vi "movimento.vi"(9 "Condição de parada":bool=TRUE, 10 "Motor speed":i32=60, 11 "Direção":T1(ring)) -> ()   [LabVIEW 2016]
uses:
  <vilib>/NXT/Block Support/NXT_InputPort.ctl
  <vilib>/NXT/Block Support/NXT_OutputPort.ctl
  <vilib>/NXT/Dual Mode Library/Sensors/EV3_Gyro_Reset.vi
  <vilib>/NXT/Dual Mode Library/Sensors/EV3_Gyro_Angle.vi
  <vilib>/NXT/NXTIO Xnodes/NXTIONodeSubVIs/NXTMoveMotors.vi
  <vilib>/NXT/NXTIO Xnodes/NXTIONodeSubVIs/NXTStopMotors.vi
  <vilib>/NXT/Subs/LVHSConnector.ctl
  <vilib>/NXT/NXTIO Xnodes/AddressXNode/NXTIOAddress.xnode
  <vilib>/NXT/NXTIO Xnodes/NXTIOXNode/NXTIO.xnode
  <vilib>/NXT/LegoClasses/BrickReference/BrickReference.lvclass
panel:
  out "Degrees":sgl
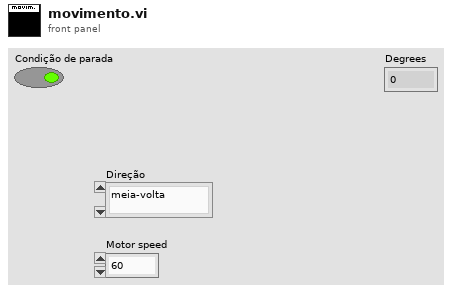
[diagram p1: front panel]
types:
  T1 = enum16{"meia-volta", "esquerda", "direita", "frente"}
  T2 = typedef "NXT_InputPort.ctl" = u32
  T3 = typedef "LVHSConnector.ctl" = refnum<class "BrickReference.lvclass">
  T4 = typedef "NXT_OutputPort.ctl" = u8
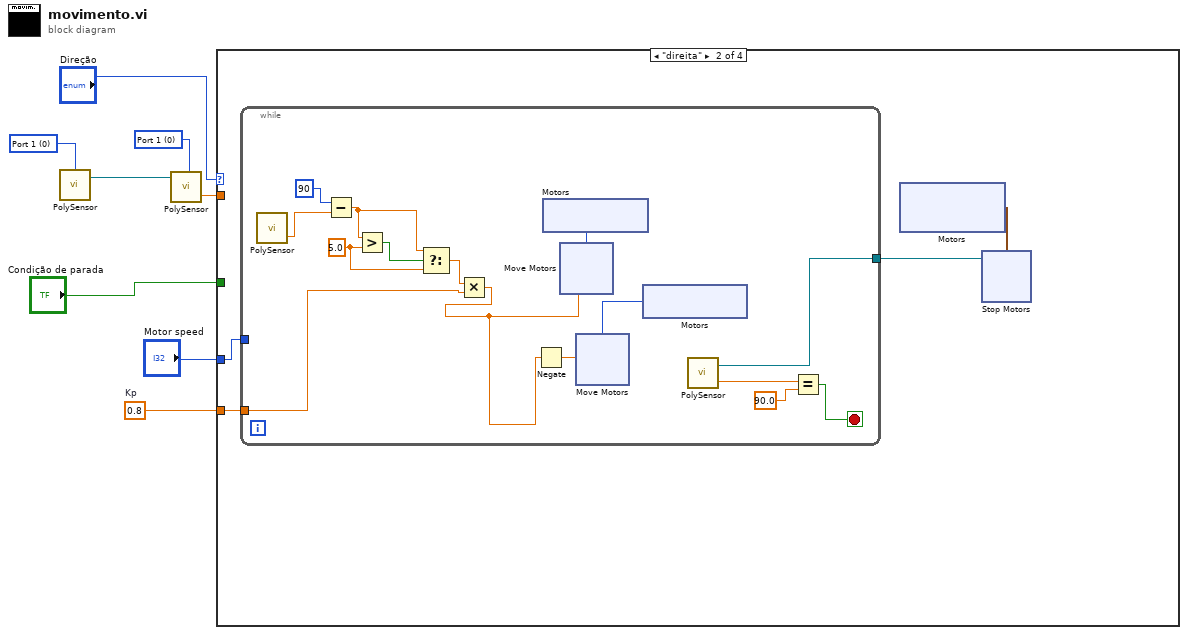
[diagram p0: block diagram]
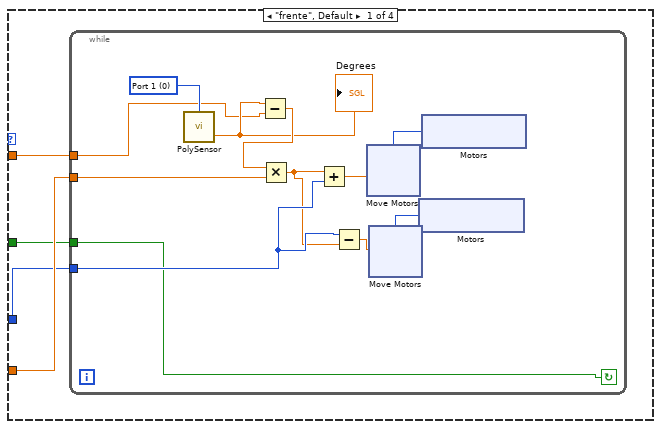
[diagram p2: hidden frame]
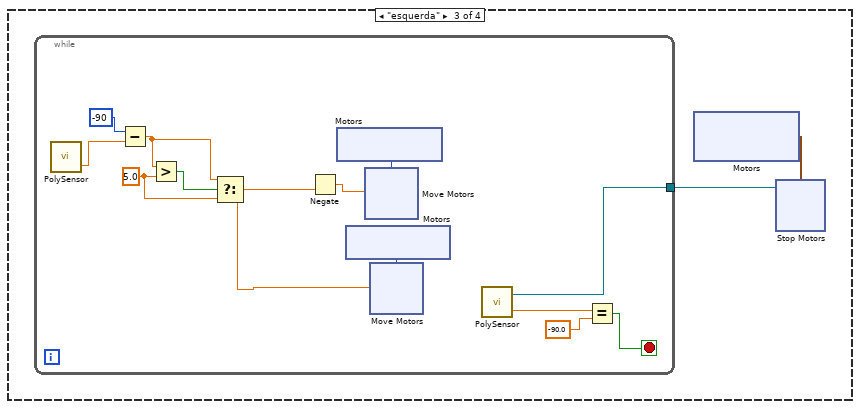
[diagram p3: hidden frame]
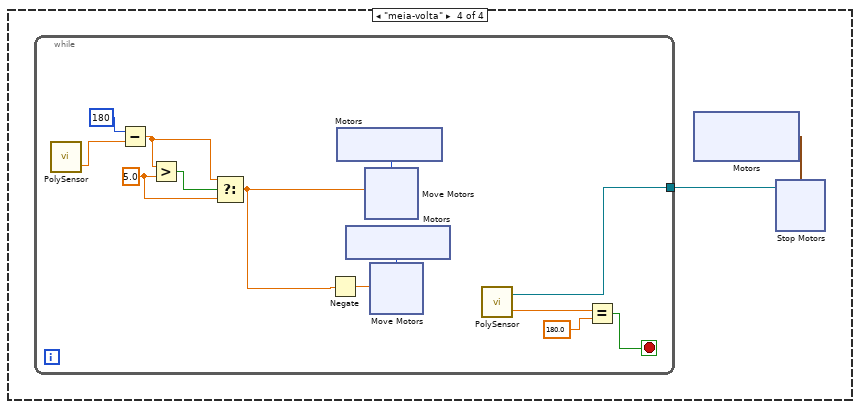
[diagram p4: hidden frame]
diagram:
  w3 = T2 0 items=["Port 1", "Port 2", "Port 3", "Port 4"] ("Port (Port 1)")
  w5 = T2 0 items=["Port 1", "Port 2", "Port 3", "Port 4"] ("Port (Port 1)")
  w8 = 0.8  # Kp
  n1 = call-poly <vilib>:"PolySensor.vi"("Port (Port 1)"=w3) -> ("NXT/EV3"=w4:T3)  [unwired: 3 in]
  n2 = call-poly <vilib>:"PolySensor.vi"("NXT/EV3"=w4, "Port (Port 1)"=w5) -> ("Degrees"=w6:sgl)  [unwired: 1 in, 1 out]
  n3 = case shown="\"direita\"" "Direção" {
    tunnel: w8 -> [w12 w41 _ _]
    tunnel: "Motor speed" -> [w11 w44 _ _]
    tunnel: w6 -> [w10 _ _ _]
    tunnel: "Condição de parada" -> [w9 _ _ _]
    frame "frente", Default {
      n4 = while {
        tunnel: w12 -> [w21]
        tunnel: w11 -> [w20]
        tunnel: w10 -> [w15]
        tunnel: w9 -> [w13]
        stop <- w13 continue-if-true
        w18 = T2 0 items=["Port 1", "Port 2", "Port 3", "Port 4"] ("Port (Port 1)")
        n5 = call-poly <vilib>:"PolySensor.vi"("Port (Port 1)"=w18) -> ("Degrees"=w16:sgl)  [unwired: 2 in, 1 out]
        "Degrees" <- w16
        n6 = Subtract(x=w16, y=w15) -> (x-y=w17:sgl)
        n7 = Multiply(x=w17, y=w21) -> (x*y=w19:dbl)
        n8 = Add(x=w19, y=w20) -> (x+y=w22:dbl)
        n9 = Subtract(x=w20, y=w19) -> (x-y=w14:dbl)
        n10 = xnode "Motors"() -> ("Motor"=w23:T4)
        n11 = xnode "Move Motors"("Power/Speed 1"=w14, "Motors"=w23) -> ()  [unwired: 1 in, 1 out]
        n12 = xnode "Motors"() -> ("Motor"=w24:T4)
        n13 = xnode "Move Motors"("Power/Speed 1"=w22, "Motors"=w24) -> ()  [unwired: 1 in, 1 out]
      }
    }
    frame "direita" {
      n14 = while {
        tunnel: w44 -> [_]
        tunnel: [w59] -> w42
        tunnel: w41 -> [w52]
        stop <- w60 stop-if-true
        w54 = sgl 5.0 ("y")
        n15 = call-poly <vilib>:"PolySensor.vi"() -> ("Degrees"=w57:sgl)  [unwired: 3 in, 1 out]
        n16 = Subtract(x=90, y=w57) -> (x-y=w55:sgl)
        n17 = Greater?(x=w55, y=w54) -> (0:w56:bool)
        n18 = Select(t=w55, s=w56, f=w54) -> (s? t:f=w53:sgl)
        n19 = Multiply(x=w53, y=w52) -> (x*y=w51:dbl)
        n20 = Negate(x=w51) -> (-x=w61:dbl)
        n21 = xnode "Motors"() -> ("Motor"=w63:T4)
        n22 = xnode "Move Motors"("Power/Speed 1"=w51, "Motors"=w63) -> ()  [unwired: 1 in, 1 out]
        n23 = xnode "Motors"() -> ("Motor"=w62:T4)
        n24 = xnode "Move Motors"("Power/Speed 1"=w61, "Motors"=w62) -> ()  [unwired: 1 in, 1 out]
        n25 = call-poly <vilib>:"PolySensor.vi"() -> ("Degrees"=w65:sgl, "NXT/EV3"=w59:T3)  [unwired: 3 in]
        n26 = Equal?(x=w65, y=sgl 90.0) -> (x = y?=w60:bool)
      }
      n27 = xnode "Motors"() -> ("Motor"=w43:cluster{"Port":T4, "Port":T4})
      n28 = xnode "Stop Motors"("Motors"=w43, "NXT/EV3"=w42) -> ()  [unwired: 1 out]
    }
    frame "esquerda" {
      n29 = while {
        tunnel: [w97] -> w82
        stop <- w98 stop-if-true
        w92 = sgl 5.0 ("y")
        n30 = call-poly <vilib>:"PolySensor.vi"() -> ("Degrees"=w95:sgl)  [unwired: 3 in, 1 out]
        n31 = Subtract(x=-90, y=w95) -> (x-y=w93:sgl)
        n32 = Greater?(x=w93, y=w92) -> (0:w94:bool)
        n33 = Select(t=w93, s=w94, f=w92) -> (s? t:f=w91:sgl)
        n34 = Negate(x=w91) -> (-x=w90:sgl)
        n35 = xnode "Motors"() -> ("Motor"=w100:T4)
        n36 = xnode "Motors"() -> ("Motor"=w99:T4)
        n37 = xnode "Move Motors"("Power/Speed 1"=w90, "Motors"=w100) -> ()  [unwired: 1 in, 1 out]
        n38 = xnode "Move Motors"("Power/Speed 1"=w91, "Motors"=w99) -> ()  [unwired: 1 in, 1 out]
        n39 = call-poly <vilib>:"PolySensor.vi"() -> ("Degrees"=w102:sgl, "NXT/EV3"=w97:T3)  [unwired: 3 in]
        n40 = Equal?(x=w102, y=sgl -90.0) -> (x = y?=w98:bool)
      }
      n41 = xnode "Motors"() -> ("Motor"=w83:cluster{"Port":T4, "Port":T4})
      n42 = xnode "Stop Motors"("Motors"=w83, "NXT/EV3"=w82) -> ()  [unwired: 1 out]
    }
    frame "meia-volta" {
      n43 = while {
        tunnel: [w133] -> w119
        stop <- w134 stop-if-true
        w128 = sgl 5.0 ("y")
        n44 = call-poly <vilib>:"PolySensor.vi"() -> ("Degrees"=w131:sgl)  [unwired: 3 in, 1 out]
        n45 = Subtract(x=180, y=w131) -> (x-y=w129:sgl)
        n46 = Greater?(x=w129, y=w128) -> (0:w130:bool)
        n47 = Select(t=w129, s=w130, f=w128) -> (s? t:f=w127:sgl)
        n48 = Negate(x=w127) -> (-x=w135:sgl)
        n49 = xnode "Motors"() -> ("Motor"=w137:T4)
        n50 = xnode "Motors"() -> ("Motor"=w136:T4)
        n51 = xnode "Move Motors"("Power/Speed 1"=w127, "Motors"=w137) -> ()  [unwired: 1 in, 1 out]
        n52 = xnode "Move Motors"("Power/Speed 1"=w135, "Motors"=w136) -> ()  [unwired: 1 in, 1 out]
        n53 = call-poly <vilib>:"PolySensor.vi"() -> ("Degrees"=w139:sgl, "NXT/EV3"=w133:T3)  [unwired: 3 in]
        n54 = Equal?(x=w139, y=sgl 180.0) -> (x = y?=w134:bool)
      }
      n55 = xnode "Motors"() -> ("Motor"=w120:cluster{"Port":T4, "Port":T4})
      n56 = xnode "Stop Motors"("Motors"=w120, "NXT/EV3"=w119) -> ()  [unwired: 1 out]
    }
  }
